vi "Excel Find Application Directory.vi"(11 "error in":errorcluster) -> (4 "application directory":path, 15 "error out":errorcluster)   [LabVIEW 2010, in "NI_ReportGenerationToolkit.lvlib"]
uses:
  <vilib>/addons/_office/NI_ReportGenerationToolkit.lvlib
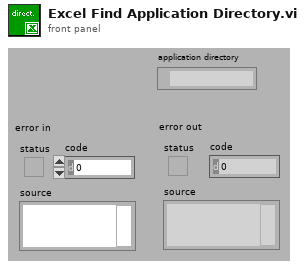
[diagram p1: front panel]
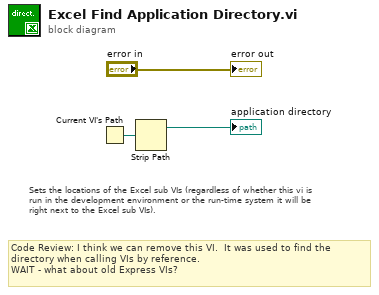
[diagram p0: block diagram]
diagram:
  # "Code Review: I think we can remove this VI.  It was used to find the directory when calling VIs by reference.\nWAIT - what about old Express VIs?"
  # "Sets the locations of the Excel sub VIs (regardless of whether this vi is run in the development environment or the run-time system it will be right next to the Excel sub VIs)."
  n1 = Current VI's Path() -> (path=w3:path)
  n2 = Strip Path(path=w3) -> (stripped path=→"application directory":path)  [unwired: 1 out]
  "error out" <- "error in"
